vi "mcp&phosvol.vi"() -> ()   [LabVIEW 2014, in "Panels.lvlib"]
uses:
  Panels.lvlib
  CSlibraries-extern/DimLVEvent/DimIndicators/DimIndicators.lvlib
  CSCore/CSSystem/CoreLib/CoreLib.lvlib
  CSlibraries/UtilityLib/UtilityLib.valueStatus.ctl
  CSlibraries/UtilityLib/UtilityLib.lvlib
  CSlibraries-extern/DimLVEvent/LVDimInterface/LVDimInterface.lvlib
  Instance           1 19Saved   mcp&phosvol .vi
  CSlibraries-extern/DimLVEvent/DimIndicators/DimIndicators.numericArrayType.ctl
  CSlibraries-extern/DimLVEvent/DimIndicators/DimIndicators.anyType.ctl
  CSlibraries-extern/DimLVEvent/DimIndicators/DimIndicators.numericType.ctl
panel:
  in  "MPC_Collector_SetValueInfoData":T1={"data"=[0.0, 2200.0, -1.0], "no link"=FALSE, "quality"=0, "timeStamp"=3270208308.169}
  in  "CEM_Plate_SetValueInfoData":T1={"data"=[0.0, 2200.0, -1.0], "no link"=FALSE, "quality"=0, "timeStamp"=3270208308.169}
  in  "MPC_Collector_SetData":T1={"data"=[0.0, 0.0, 0.0, 0.0], "no link"=FALSE, "quality"=1, "timeStamp"=3270208307.575}
  in  "CEM_Plate_SetData":T1={"data"=[0.0, 0.0, 0.0, 0.0], "no link"=FALSE, "quality"=1, "timeStamp"=3270208307.575}
  in  "Daly_Collector_MonData":T2={"data"=inf, "no link"=FALSE, "quality"=1, "timeStamp"=3270208308.169}
  in  "CEM_Plate_MonData":T2={"data"=inf, "no link"=FALSE, "quality"=1, "timeStamp"=3270208308.169}
  in  "Daly_Collector":bool
  out "Daly_Collector_Mon":dbl=inf format="%.4f"
  in  "CEM_Plate":bool
  out "CEM_Plate_Mon":dbl=inf format="%.4f"
  in  "BOB3_PHO_SetValueInfoData":T1={"data"=[0.0, 2000.0, -1.0], "no link"=FALSE, "quality"=0, "timeStamp"=3270208308.169}
  in  "SetFileLocation_Data":T3={"data"="NOLINK", "no link"=TRUE, "quality"=-1, "timeStamp"=0.0}
  in  "BOB1_MCP":bool
  in  "BOB1_Pho":bool
  in  "BOB6MCPin_MonData":T2={"data"=32767.0, "no link"=FALSE, "quality"=1, "timeStamp"=3270208308.169}
  in  "BOB3MCPout_MonData":T2={"data"=32767.0, "no link"=FALSE, "quality"=1, "timeStamp"=3270208308.169}
  in  "BOB1BETAout_MonData":T2={"data"=32767.0, "no link"=FALSE, "quality"=1, "timeStamp"=3270208308.169}
  in  "BOB2MCPin_MonData":T2={"data"=32767.0, "no link"=FALSE, "quality"=1, "timeStamp"=3270208308.169}
  in  "BOB1BETAin_MonData":T2={"data"=32767.0, "no link"=FALSE, "quality"=1, "timeStamp"=3270208308.153}
  in  "BOB2MCPout_MonData":T2={"data"=32767.0, "no link"=FALSE, "quality"=1, "timeStamp"=3270208308.153}
  in  "BOB3MCPin_MonData":T2={"data"=32767.0, "no link"=FALSE, "quality"=1, "timeStamp"=3270208308.169}
  in  "BOB6MCPout_MonData":T2={"data"=32767.0, "no link"=FALSE, "quality"=1, "timeStamp"=3270208308.169}
  in  "BOB5MCPin_MonData":T2={"data"=32767.0, "no link"=FALSE, "quality"=1, "timeStamp"=3270208308.169}
  in  "BOB5MCPout_MonData":T2={"data"=32767.0, "no link"=FALSE, "quality"=1, "timeStamp"=3270208308.169}
  in  "BOB4MCPin_MonData":T2={"data"=32767.0, "no link"=FALSE, "quality"=1, "timeStamp"=3270208308.169}
  in  "BOB4MCPout_MonData":T2={"data"=32767.0, "no link"=FALSE, "quality"=1, "timeStamp"=3270208308.169}
  out "BOB6MCPin_Mon":bool
  out "BOB6MCPout_Mon":bool
  out "BOB5MCPin_Mon":bool
  out "BOB5MCPout_Mon":bool
  out "BOB4MCPin_Mon":bool
  out "BOB4MCPin_Mon":bool
  out "BOB3MCPin_Mon":bool
  out "BOB3MCPout_Mon":bool
  out "BOB2MCPin_Mon":bool
  out "BOB2MCPout_Mon":bool
  out "BOB1BETAin_Mon":bool
  out "BOB1BETAout_Mon":bool
  in  "SetFileLocation":path=path "\\\\intranet\\Files/projects/lebit/Data Exchange/data/MCP&PhosVolControl"
  in  "BOB6_MCP_SetValueInfoData":T1={"data"=[0.0, 2200.0, -1.0], "no link"=FALSE, "quality"=0, "timeStamp"=3270208308.169}
  in  "BOB6_MCP_SetData":T1={"data"=[0.0, 0.0, 0.0, 0.0], "no link"=FALSE, "quality"=1, "timeStamp"=3270208307.575}
  in  "BOB6_MCP_MonData":T2={"data"=inf, "no link"=FALSE, "quality"=1, "timeStamp"=3270208308.169}
  in  "BOB6_MCP":bool
  in  "BOB6_Pho":bool
  in  "BOB5_MCP":bool
  in  "BOB5_Pho":bool
  in  "BOB3_MCP":bool
  in  "BOB3_Pho":bool
  in  "BOB6_Pho_SetValueInfoData":T1={"data"=[0.0, 3000.0, -1.0], "no link"=FALSE, "quality"=0, "timeStamp"=3270208308.169}
  in  "BOB6_Pho_SetData":T1={"data"=[0.0, 0.0, 0.0, 0.0], "no link"=FALSE, "quality"=1, "timeStamp"=3270208307.575}
  in  "BOB6_Pho_MonData":T2={"data"=inf, "no link"=FALSE, "quality"=1, "timeStamp"=3270208308.169}
  out "BOB2_MCP_Mon":dbl=inf format="%.4f"
  out "BOB1_MCP_Mon":dbl=inf format="%.4f"
  out "i ref out":refnum<vi>
  in  "Last Loaded File_Data":T3={"data"="NOLINK", "no link"=TRUE, "quality"=-1, "timeStamp"=0.0}
  out "FileUpToDate":bool=TRUE caption="Parameter Changed"
  in  "BOB1_MCP_SetValueInfoData":T1={"data"=[0.0, 10.0, -1.0], "no link"=FALSE, "quality"=0, "timeStamp"=3270208308.153}
  in  "BOB2_Pho_SetValueInfoData":T1={"data"=[0.0, 3000.0, -1.0], "no link"=FALSE, "quality"=0, "timeStamp"=3270208308.169}
  in  "BOB2_MCP_SetValueInfoData":T1={"data"=[0.0, 10.0, -1.0], "no link"=FALSE, "quality"=0, "timeStamp"=3270208308.169}
  in  "BOB3_MCP_SetValueInfoData":T1={"data"=[0.0, 2000.0, -1.0], "no link"=FALSE, "quality"=0, "timeStamp"=3270208308.169}
  in  "BOB4_Pho_SetValueInfoData":T1={"data"=[0.0, 3000.0, -1.0], "no link"=FALSE, "quality"=0, "timeStamp"=3270208308.169}
  in  "BOB4_MCP_SetValueInfoData":T1={"data"=[0.0, 2000.0, -1.0], "no link"=FALSE, "quality"=0, "timeStamp"=3270208308.169}
  in  "BOB5_Pho_SetValueInfoData":T1={"data"=[0.0, 3000.0, -1.0], "no link"=FALSE, "quality"=0, "timeStamp"=3270208308.153}
  in  "BOB5_MCP_SetValueInfoData":T1={"data"=[0.0, 2000.0, -1.0], "no link"=FALSE, "quality"=0, "timeStamp"=3270208308.169}
  in  "BOB1_Pho_SetValueInfoData":T1={"data"=[0.0, 10.0, -1.0], "no link"=FALSE, "quality"=0, "timeStamp"=3270208308.169}
  in  "BOB1_Pho_SetData":T1={"data"=[0.0, 0.0, 0.0, 0.0], "no link"=FALSE, "quality"=1, "timeStamp"=3270208307.575}
  in  "BOB5_Pho_SetData":T1={"data"=[0.0, 0.0, 0.0, 0.0], "no link"=FALSE, "quality"=1, "timeStamp"=3270208307.575}
  in  "BOB4_MCP_SetData":T1={"data"=[0.0, 0.0, 0.0, 0.0], "no link"=FALSE, "quality"=1, "timeStamp"=3270208307.575}
  in  "BOB4_Pho_SetData":T1={"data"=[0.0, 0.0, 0.0, 0.0], "no link"=FALSE, "quality"=1, "timeStamp"=3270208307.575}
  in  "BOB3_MCP_SetData":T1={"data"=[0.0, 0.0, 0.0, 0.0], "no link"=FALSE, "quality"=1, "timeStamp"=3270208307.575}
  in  "BOB3_Pho_SetData":T1={"data"=[0.0, 0.0, 0.0, 0.0], "no link"=FALSE, "quality"=1, "timeStamp"=3270208307.591}
  in  "BOB2_MCP_SetData":T1={"data"=[0.0, 0.0, 0.0, 0.0], "no link"=FALSE, "quality"=1, "timeStamp"=3270208307.575}
  in  "BOB2_Pho_SetData":T1={"data"=[0.0, 0.0, 0.0, 0.0], "no link"=FALSE, "quality"=1, "timeStamp"=3270208307.575}
  in  "BOB1_MCP_SetData":T1={"data"=[0.0, 0.0, 0.0, 0.0], "no link"=FALSE, "quality"=1, "timeStamp"=3270208307.575}
  in  "BOB5_MCP_SetData":T1={"data"=[0.0, 0.0, 0.0, 0.0], "no link"=FALSE, "quality"=1, "timeStamp"=3270208307.575}
  out "Last Loaded File":string
  in  "BOB5_MCP_MonData":T2={"data"=inf, "no link"=FALSE, "quality"=1, "timeStamp"=3270208308.169}
  in  "BOB5_Pho_MonData":T2={"data"=inf, "no link"=FALSE, "quality"=1, "timeStamp"=3270208308.169}
  in  "BOB4_MCP_MonData":T2={"data"=inf, "no link"=FALSE, "quality"=1, "timeStamp"=3270208308.169}
  in  "BOB4_Pho_MonData":T2={"data"=inf, "no link"=FALSE, "quality"=1, "timeStamp"=3270208308.169}
  in  "BOB3_MCP_MonData":T2={"data"=inf, "no link"=FALSE, "quality"=1, "timeStamp"=3270208308.169}
  in  "BOB3_Pho_MonData":T2={"data"=inf, "no link"=FALSE, "quality"=1, "timeStamp"=3270208308.169}
  in  "BOB2_MCP_MonData":T2={"data"=inf, "no link"=FALSE, "quality"=1, "timeStamp"=3270208308.153}
  in  "BOB2_Pho_MonData":T2={"data"=inf, "no link"=FALSE, "quality"=1, "timeStamp"=3270208308.153}
  in  "BOB1_MCP_MonData":T2={"data"=inf, "no link"=FALSE, "quality"=1, "timeStamp"=3270208308.169}
  in  "BOB1_Pho_MonData":T2={"data"=inf, "no link"=FALSE, "quality"=1, "timeStamp"=3270208308.169}
  out "BOB3_MCP_Mon":dbl=inf format="%.4f"
  out "BOB2_Pho_Mon":dbl=inf format="%.4f"
  out "BOB6_MCP_Mon":dbl=inf format="%.4f"
  out "BOB4_Pho_Mon":dbl=inf format="%.4f"
  out "BOB3_Pho_Mon":dbl=inf format="%.4f"
  out "BOB1_Pho_Mon":dbl=inf format="%.4f"
  out "BOB5_Pho_Mon":dbl=inf format="%.4f"
  out "BOB4_MCP_Mon":dbl=inf format="%.4f"
  out "BOB5_MCP_Mon":dbl=inf format="%.4f"
  out "BOB6_Pho_Mon":dbl=inf format="%.4f"
  # "Parameter changed, data file is no longer up-to-date."
  # "BOB2_Pho"
  # "BOB4_Pho"
  # "BOB2_MCP"
  # "BOB4_MCP"
  # "IN"
  # "OUT"
  # "IN"
  # "OUT"
  # "IN"
  # "OUT"
  # "IN"
  # "OUT"
  # "IN"
  # "OUT"
  # "IN"
  # "OUT"
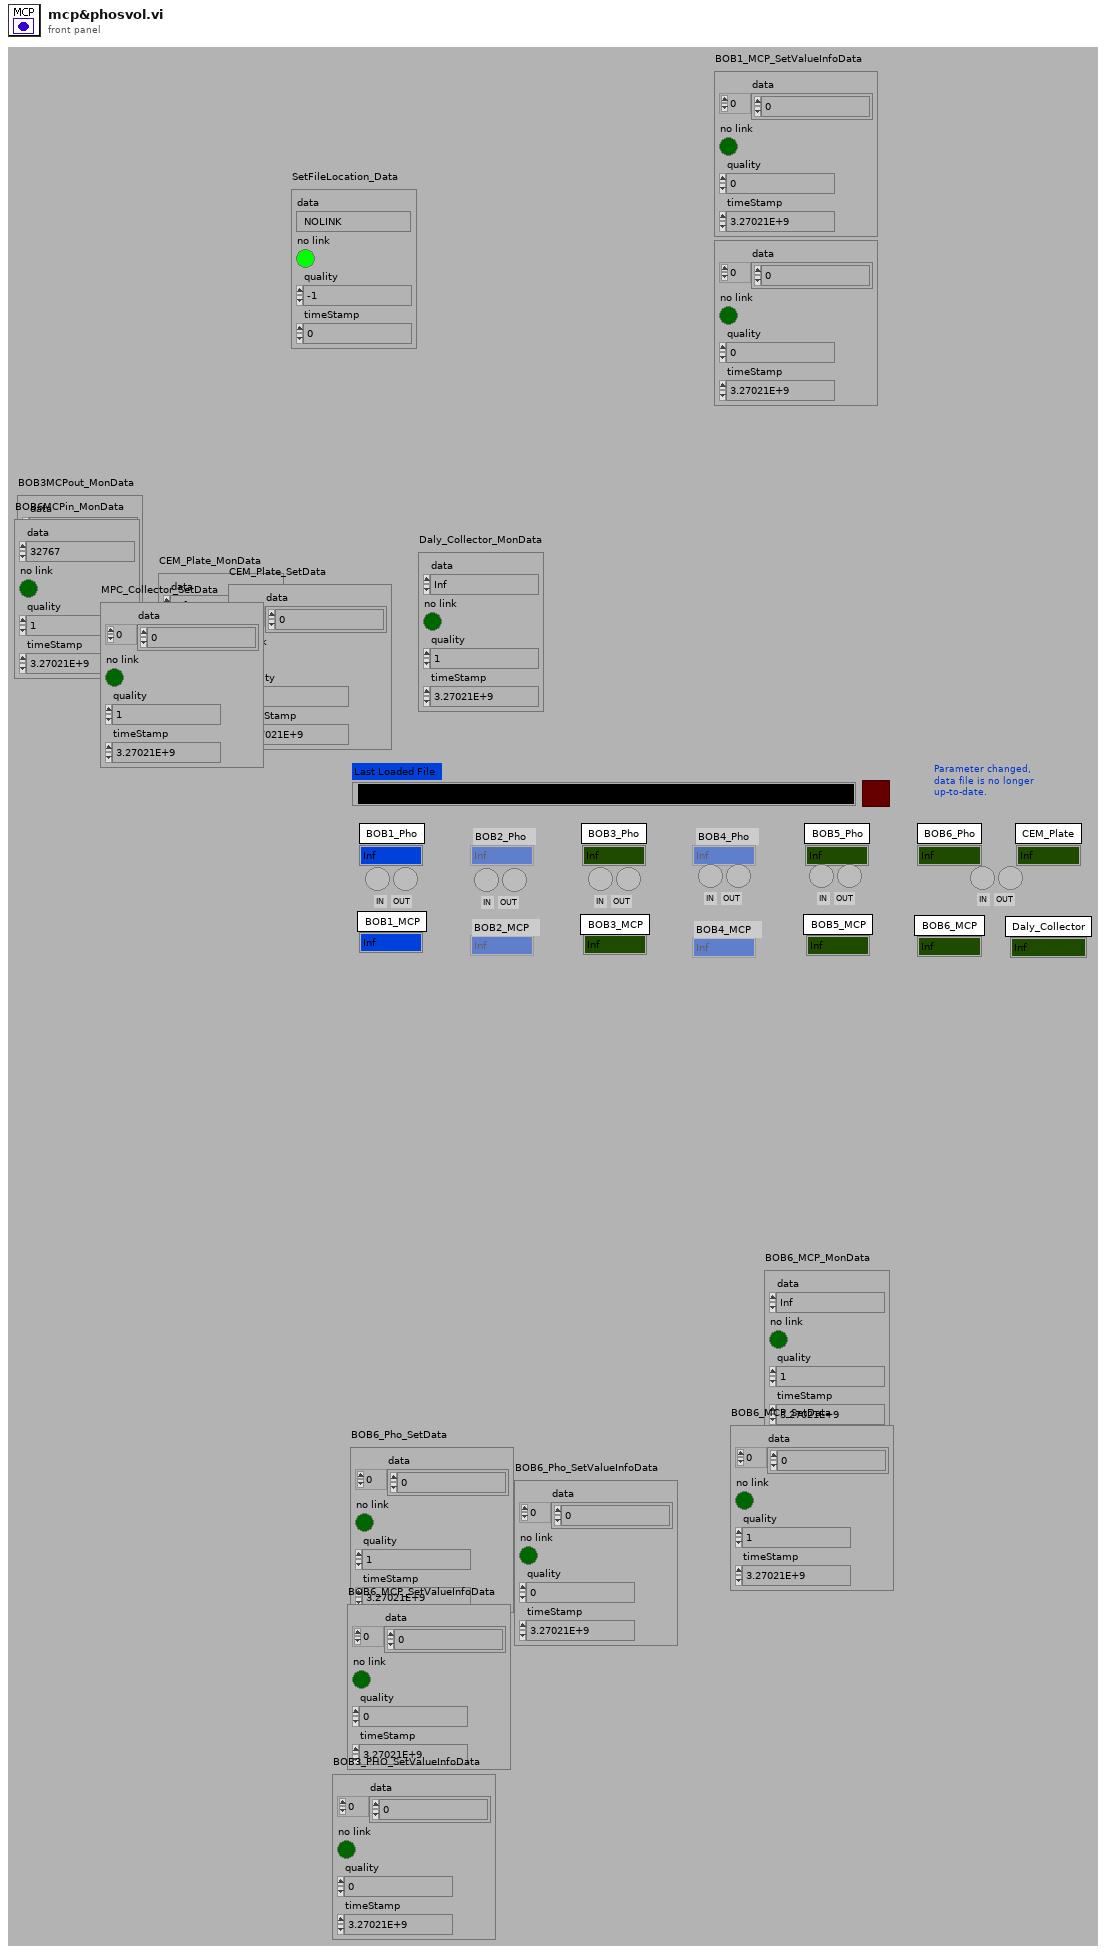
[diagram p1: front panel]
types:
  T1 = typedef "DimIndicators.lvlib/DimIndicators.numericArrayType.ctl" = cluster{"data":dbl[], "no link":bool, "quality":i32, "timeStamp":dbl}
  T2 = typedef "DimIndicators.lvlib/DimIndicators.numericType.ctl" = cluster{"data":dbl, "no link":bool, "quality":i32, "timeStamp":dbl}
  T3 = typedef "DimIndicators.lvlib/DimIndicators.anyType.ctl" = cluster{"data":string, "no link":bool, "quality":i32, "timeStamp":dbl}
  T4 = typedef "UtilityLib.lvlib/UtilityLib.valueStatus.ctl" = enum16{"no info available", "stand by/off", "on", "warning", "alarm/malfunction", "not implemented", "user action required", "important information", "system default", "control default", "indicator default", "button default"}
  T5 = cluster{"data":string, "no link":bool, "quality":i32, "timeStamp":dbl}
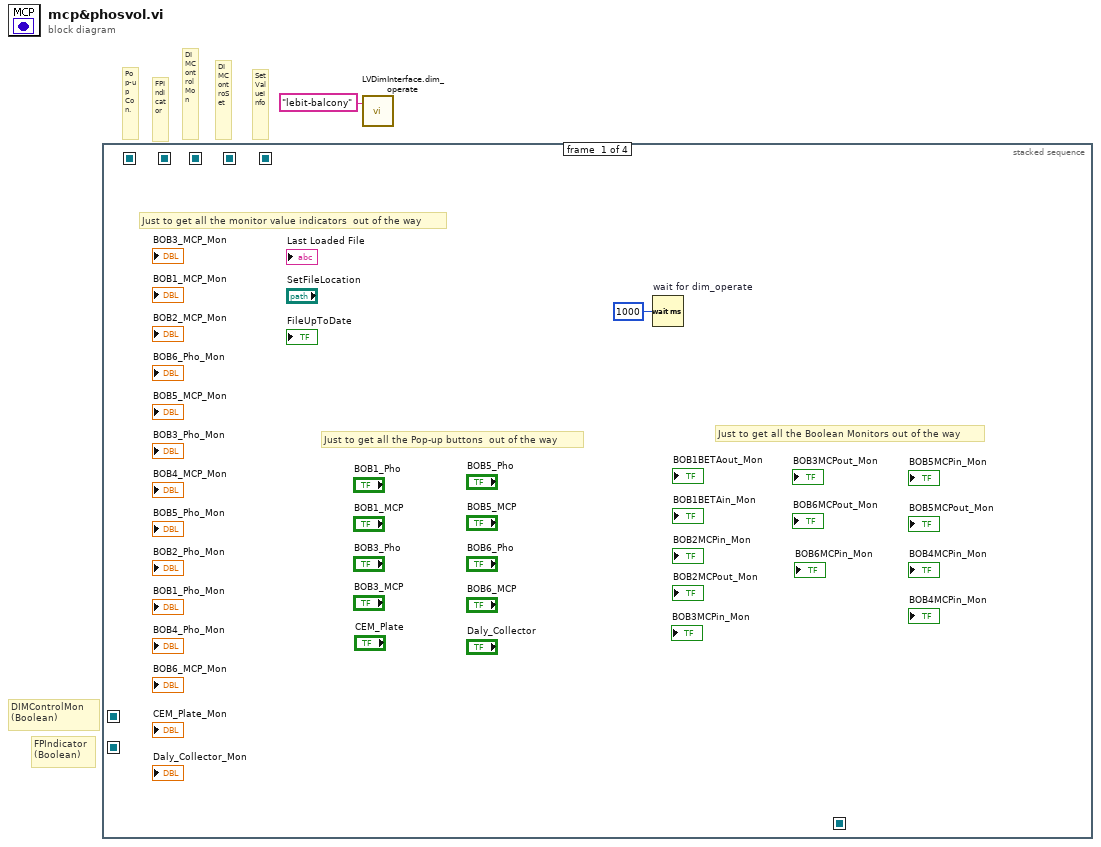
[diagram p0: block diagram]
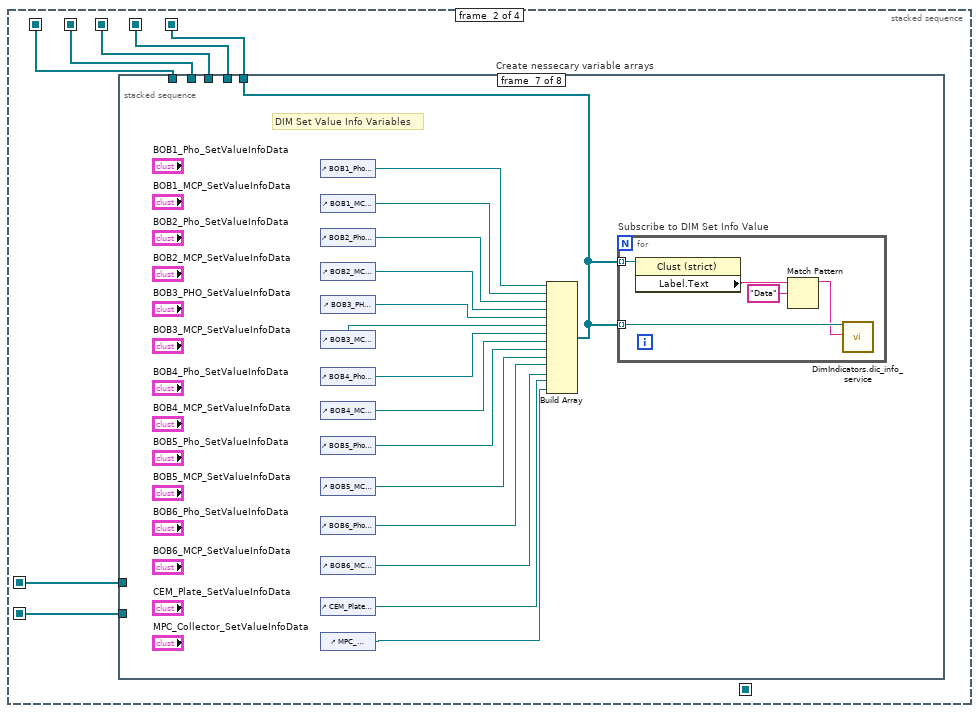
[diagram p2: hidden frame]
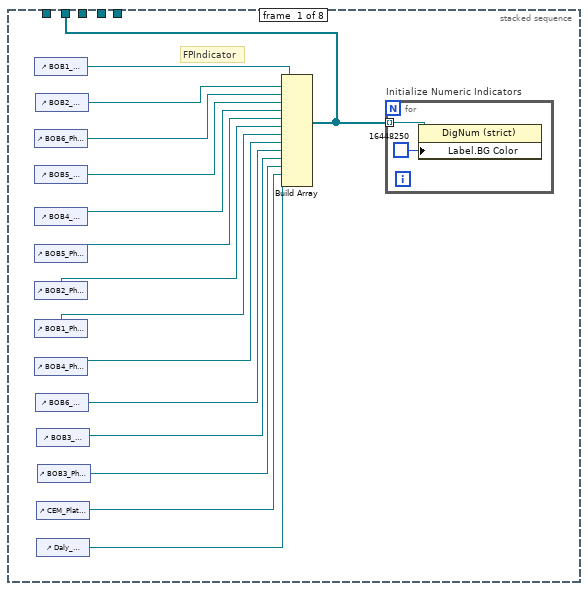
[diagram p3: hidden frame]
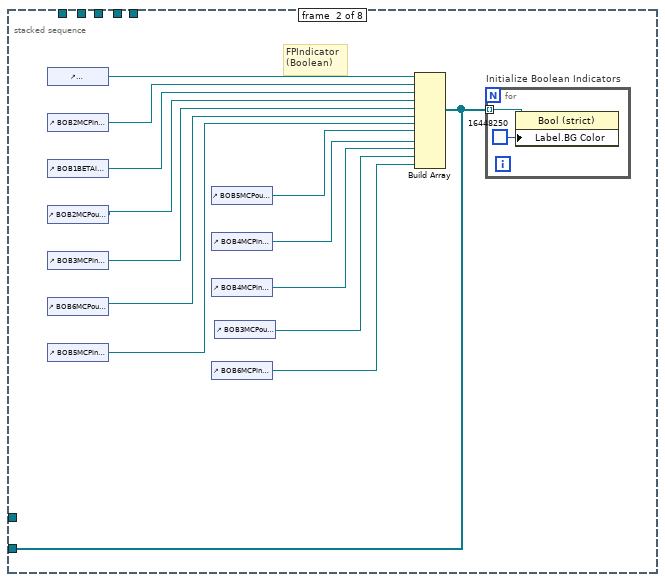
[diagram p4: hidden frame]
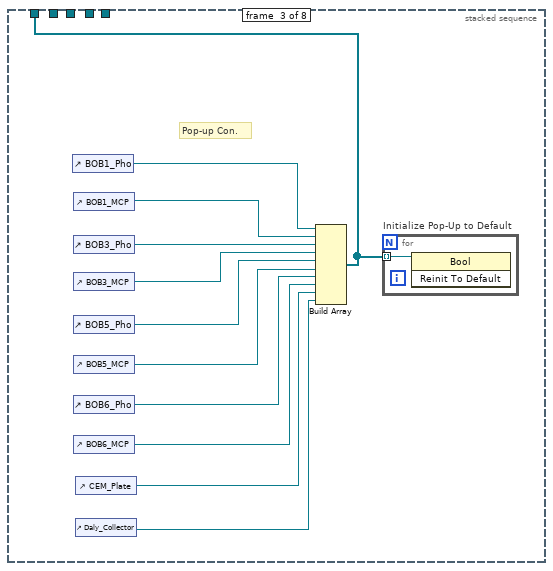
[diagram p5: hidden frame]
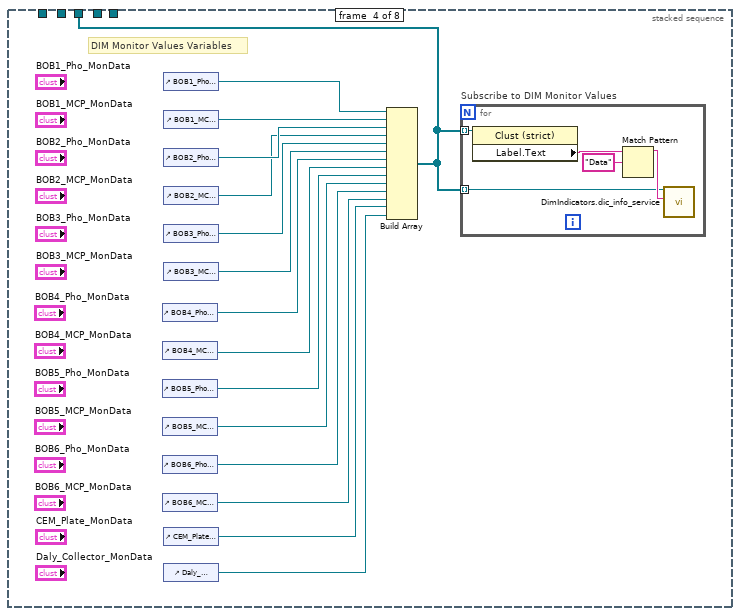
[diagram p6: hidden frame]
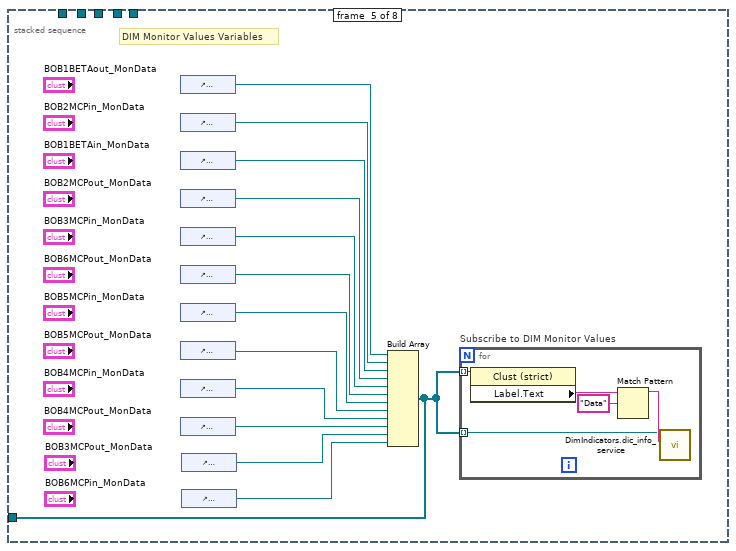
[diagram p7: hidden frame]
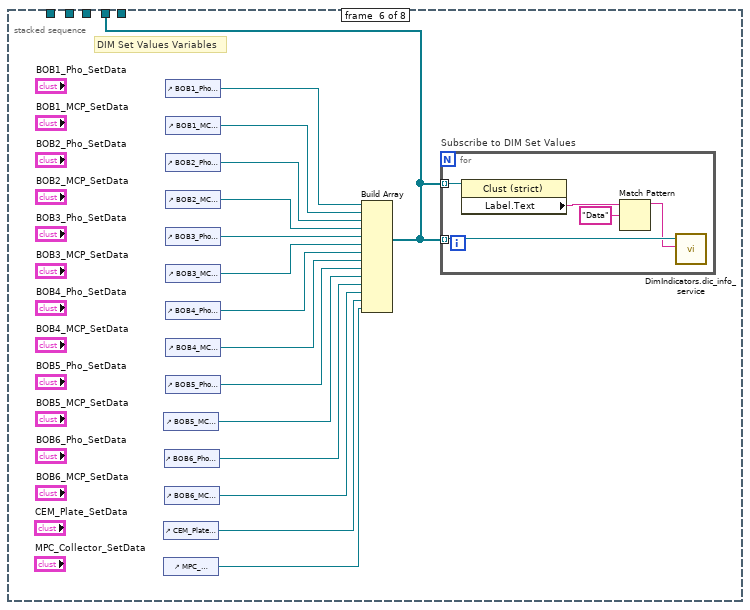
[diagram p8: hidden frame]
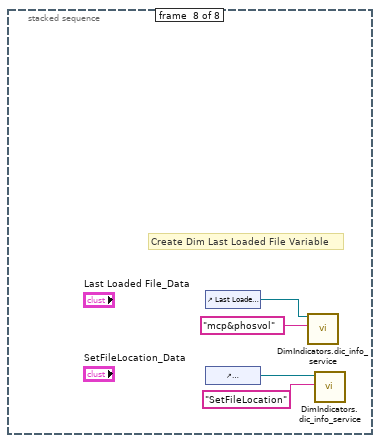
[diagram p9: hidden frame]
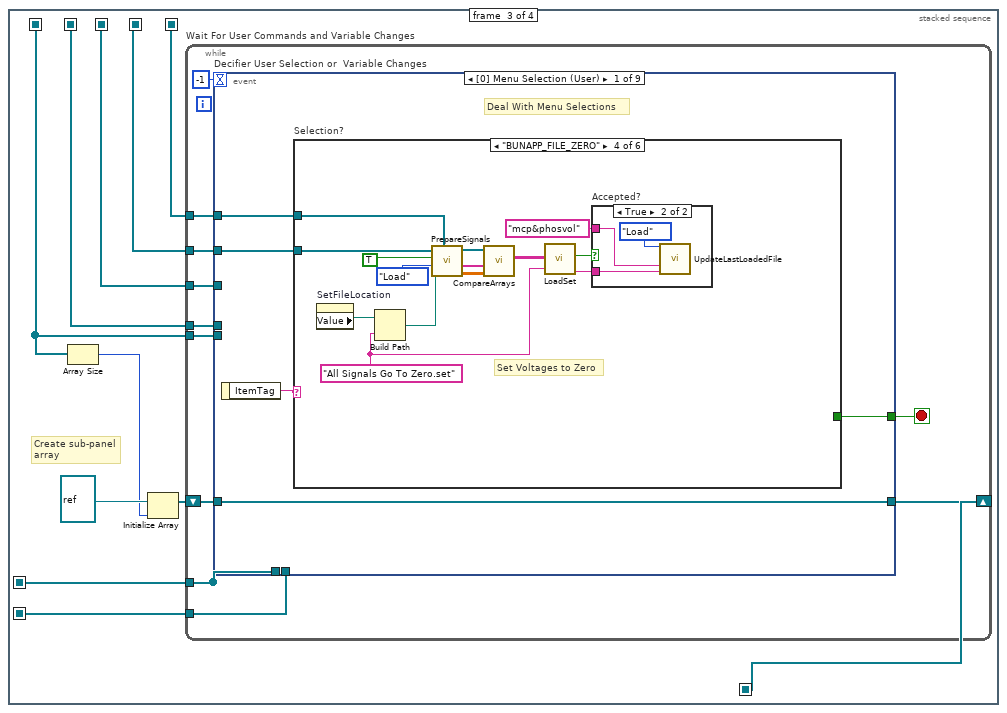
[diagram p10: hidden frame]
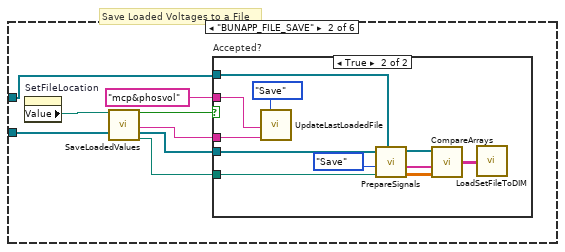
[diagram p12: hidden frame]
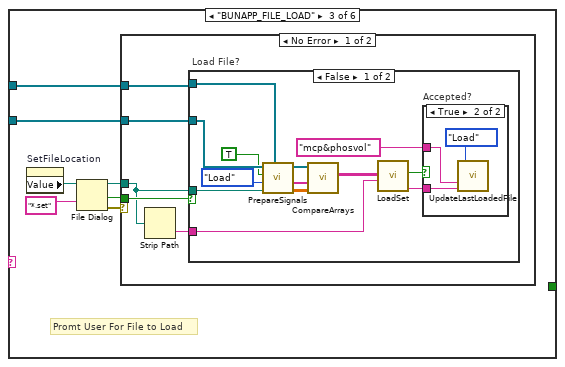
[diagram p14: hidden frame]
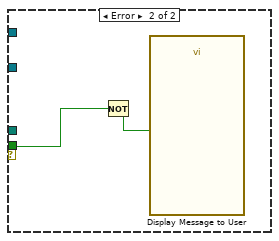
[diagram p17: hidden frame]
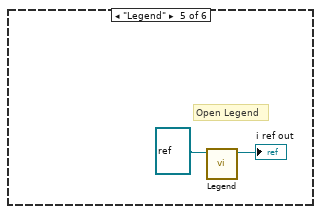
[diagram p19: hidden frame]
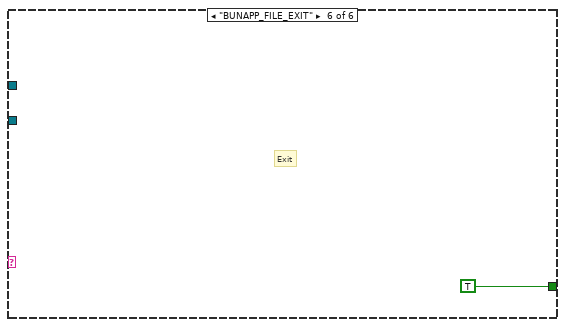
[diagram p20: hidden frame]
diagram:
  # "FPIndicator\n(Boolean)"
  # "DIMControlMon\n(Boolean)"
  # "Pop-up Con."
  # "SetValueInfo"
  # "DIMControSet"
  # "DIMControlMon"
  # "FPIndicator"
  n1 = stacked-sequence {
    seq-local: [_ w9 _ _] -> [_ _ w143 _]
    seq-local: [_ w4 _ _] -> [_ _ w146 w375]
    seq-local: [_ _ w141 _] -> [_ _ _ w374]
    seq-local: [_ w5 _ _] -> [_ _ w140 w373]
    seq-local: [_ w3 _ _] -> [_ _ w139 w372]
    seq-local: [_ w7 _ _] -> [_ _ w138 _]
    seq-local: [_ w8 _ _] -> [_ _ w136 _]
    seq-local: [_ w6 _ _] -> [_ _ w137 w371]
    frame #0 {
      # "Just to get all the Boolean Monitors out of the way"
      # "Just to get all the Pop-up buttons  out of the way"
      # "Just to get all the monitor value indicators  out of the way"
      n2 = Wait (ms) "wait for dim_operate"(milliseconds to wait=u32 1000) -> ()  [unwired: 1 out]
    }
    frame #1 {
      # "Arrange references to all monitor-value related buttons into an array."
      n3 = stacked-sequence "Create nessecary variable arrays" {
        tunnel: [w12 _ _ _ _ _ _ _] -> w9
        tunnel: [_ w27 _ _ _ _ _ _] -> w8
        tunnel: [_ _ w44 _ _ _ _ _] -> w7
        tunnel: [_ _ _ w56 _ _ _ _] -> w4
        tunnel: [_ _ _ _ w74 _ _ _] -> w6
        tunnel: [_ _ _ _ _ w94 _ _] -> w5
        tunnel: [_ _ _ _ _ _ w116 _] -> w3
        frame #0 {
          # "FPIndicator"
          n4 = control-ref of="BOB1_MCP_Mon"() -> (w18:refnum<vi>)
          n5 = control-ref of="BOB6_Pho_Mon"() -> (w15:refnum<vi>)
          n6 = control-ref of="BOB5_MCP_Mon"() -> (w16:refnum<vi>)
          n7 = control-ref of="BOB4_MCP_Mon"() -> (w24:refnum<vi>)
          n8 = control-ref of="BOB5_Pho_Mon"() -> (w23:refnum<vi>)
          n9 = control-ref of="BOB2_Pho_Mon"() -> (w22:refnum<vi>)
          n10 = control-ref of="BOB1_Pho_Mon"() -> (w21:refnum<vi>)
          n11 = control-ref of="BOB4_Pho_Mon"() -> (w20:refnum<vi>)
          n12 = control-ref of="BOB2_MCP_Mon"() -> (w14:refnum<vi>)
          n13 = control-ref of="BOB6_MCP_Mon"() -> (w19:refnum<vi>)
          n14 = control-ref of="BOB3_MCP_Mon"() -> (w17:refnum<vi>)
          n15 = control-ref of="CEM_Plate_Mon"() -> (w11:refnum<vi>)
          n16 = control-ref of="Daly_Collector_Mon"() -> (w10:refnum<vi>)
          n17 = control-ref of="BOB3_Pho_Mon"() -> (w13:refnum<vi>)
          n18 = Build Array(w18, w14, w15, w16, w24, w23, w22, w21, w20, w19, w17, w13, w11, w10) -> (w12:refnum<vi>[])
          n19 = for "Initialize Numeric Indicators" {
            tunnel: w12 -> [w26] mode=indexing
            n20 = property class="DigNum (strict)"(reference=w26, "Label.BG Color"=u32 16448250 ("Color Box")) -> ()  [unwired: 1 in, 2 out]
          }
        }
        frame #1 {
          # "FPIndicator\n(Boolean)"
          n21 = control-ref of="BOB1BETAout_Mon"() -> (w39:refnum<vi>)
          n22 = control-ref of="BOB2MCPin_Mon"() -> (w38:refnum<vi>)
          n23 = control-ref of="BOB1BETAin_Mon"() -> (w37:refnum<vi>)
          n24 = control-ref of="BOB2MCPout_Mon"() -> (w36:refnum<vi>)
          n25 = control-ref of="BOB3MCPin_Mon"() -> (w35:refnum<vi>)
          n26 = control-ref of="BOB6MCPout_Mon"() -> (w34:refnum<vi>)
          n27 = control-ref of="BOB5MCPin_Mon"() -> (w33:refnum<vi>)
          n28 = control-ref of="BOB5MCPout_Mon"() -> (w32:refnum<vi>)
          n29 = control-ref of="BOB4MCPin_Mon"() -> (w31:refnum<vi>)
          n30 = control-ref of="BOB4MCPin_Mon"() -> (w30:refnum<vi>)
          n31 = control-ref of="BOB6MCPin_Mon"() -> (w28:refnum<vi>)
          n32 = control-ref of="BOB3MCPout_Mon"() -> (w29:refnum<vi>)
          n33 = Build Array(w39, w38, w37, w36, w35, w34, w33, w32, w31, w30, w29, w28) -> (w27:refnum<vi>[])
          n34 = for "Initialize Boolean Indicators" {
            tunnel: w27 -> [w41] mode=indexing
            n35 = property class="Bool (strict)"(reference=w41, "Label.BG Color"=u32 16448250 ("Color Box")) -> ()  [unwired: 1 in, 2 out]
          }
        }
        frame #2 {
          # "Pop-up Con."
          n36 = control-ref of="BOB1_Pho"() -> (w46:refnum<vi>)
          n37 = control-ref of="BOB1_MCP"() -> (w45:refnum<vi>)
          n38 = control-ref of="BOB3_Pho"() -> (w52:refnum<vi>)
          n39 = control-ref of="BOB3_MCP"() -> (w51:refnum<vi>)
          n40 = control-ref of="BOB5_Pho"() -> (w50:refnum<vi>)
          n41 = control-ref of="BOB5_MCP"() -> (w49:refnum<vi>)
          n42 = control-ref of="BOB6_Pho"() -> (w48:refnum<vi>)
          n43 = control-ref of="BOB6_MCP"() -> (w47:refnum<vi>)
          n44 = control-ref of="CEM_Plate"() -> (w43:refnum<vi>)
          n45 = control-ref of="Daly_Collector"() -> (w42:refnum<vi>)
          n46 = Build Array(w46, w45, w52, w51, w50, w49, w48, w47, w43, w42) -> (w44:refnum<vi>[])
          n47 = for "Initialize Pop-Up to Default" {
            tunnel: w44 -> [w53] mode=indexing
            n48 = invoke class="Bool" method="Reinit To Default"(reference=w53) -> ()  [unwired: 2 in, 3 out]
          }
        }
        frame #3 {
          # "DIM Monitor Values Variables"
          n49 = control-ref of="BOB4_Pho_MonData"() -> (w62:refnum<vi>)
          n50 = control-ref of="BOB4_MCP_MonData"() -> (w60:refnum<vi>)
          n51 = control-ref of="BOB5_Pho_MonData"() -> (w59:refnum<vi>)
          n52 = control-ref of="BOB5_MCP_MonData"() -> (w58:refnum<vi>)
          n53 = control-ref of="BOB6_Pho_MonData"() -> (w61:refnum<vi>)
          n54 = control-ref of="BOB6_MCP_MonData"() -> (w57:refnum<vi>)
          n55 = control-ref of="BOB1_Pho_MonData"() -> (w68:refnum<vi>)
          n56 = control-ref of="BOB1_MCP_MonData"() -> (w67:refnum<vi>)
          n57 = control-ref of="BOB2_Pho_MonData"() -> (w66:refnum<vi>)
          n58 = control-ref of="BOB2_MCP_MonData"() -> (w65:refnum<vi>)
          n59 = control-ref of="BOB3_Pho_MonData"() -> (w64:refnum<vi>)
          n60 = control-ref of="BOB3_MCP_MonData"() -> (w63:refnum<vi>)
          n61 = control-ref of="CEM_Plate_MonData"() -> (w55:refnum<vi>)
          n62 = control-ref of="Daly_Collector_MonData"() -> (w54:refnum<vi>)
          n63 = Build Array(w68, w67, w66, w65, w64, w63, w62, w60, w59, w58, w61, w57, w55, w54) -> (w56:refnum<vi>[])
          n64 = for "Subscribe to DIM Monitor Values" {
            tunnel: w56 -> [w70] mode=indexing
            tunnel: w56 -> [w69] mode=indexing
            n65 = property class="Clust (strict)"(reference=w69) -> ("Label.Text"=w72:string)  [unwired: 1 in, 2 out]
            n66 = Match Pattern(string=w72, regular expression="Data") -> (before substring=w71:string)  [unwired: 1 in, 3 out]
            n67 = call "DimIndicators.dic_info_service.vi"("controlRef"=w70, "serviceName"=w71) -> ()  [unwired: 16 in, 2 out]
          }
        }
        frame #4 {
          # "DIM Monitor Values Variables"
          n68 = control-ref of="BOB1BETAout_MonData"() -> (w86:refnum<vi>)
          n69 = control-ref of="BOB2MCPin_MonData"() -> (w85:refnum<vi>)
          n70 = control-ref of="BOB1BETAin_MonData"() -> (w84:refnum<vi>)
          n71 = control-ref of="BOB2MCPout_MonData"() -> (w83:refnum<vi>)
          n72 = control-ref of="BOB3MCPin_MonData"() -> (w82:refnum<vi>)
          n73 = control-ref of="BOB6MCPout_MonData"() -> (w81:refnum<vi>)
          n74 = control-ref of="BOB5MCPin_MonData"() -> (w80:refnum<vi>)
          n75 = control-ref of="BOB5MCPout_MonData"() -> (w79:refnum<vi>)
          n76 = control-ref of="BOB4MCPin_MonData"() -> (w78:refnum<vi>)
          n77 = control-ref of="BOB4MCPout_MonData"() -> (w77:refnum<vi>)
          n78 = control-ref of="BOB3MCPout_MonData"() -> (w76:refnum<vi>)
          n79 = control-ref of="BOB6MCPin_MonData"() -> (w75:refnum<vi>)
          n80 = Build Array(w86, w85, w84, w83, w82, w81, w80, w79, w78, w77, w76, w75) -> (w74:refnum<vi>[])
          n81 = for "Subscribe to DIM Monitor Values" {
            tunnel: w74 -> [w88] mode=indexing
            tunnel: w74 -> [w87] mode=indexing
            n82 = property class="Clust (strict)"(reference=w87) -> ("Label.Text"=w90:string)  [unwired: 1 in, 2 out]
            n83 = Match Pattern(string=w90, regular expression="Data") -> (before substring=w89:string)  [unwired: 1 in, 3 out]
            n84 = call "DimIndicators.dic_info_service.vi"("controlRef"=w88, "serviceName"=w89) -> ()  [unwired: 16 in, 2 out]
          }
        }
        frame #5 {
          # "DIM Set Values Variables"
          n85 = control-ref of="BOB5_MCP_SetData"() -> (w97:refnum<vi>)
          n86 = control-ref of="CEM_Plate_SetData"() -> (w93:refnum<vi>)
          n87 = control-ref of="MPC_Collector_SetData"() -> (w92:refnum<vi>)
          n88 = control-ref of="BOB6_Pho_SetData"() -> (w96:refnum<vi>)
          n89 = control-ref of="BOB6_MCP_SetData"() -> (w95:refnum<vi>)
          n90 = control-ref of="BOB1_Pho_SetData"() -> (w106:refnum<vi>)
          n91 = control-ref of="BOB1_MCP_SetData"() -> (w105:refnum<vi>)
          n92 = control-ref of="BOB2_Pho_SetData"() -> (w104:refnum<vi>)
          n93 = control-ref of="BOB2_MCP_SetData"() -> (w103:refnum<vi>)
          n94 = control-ref of="BOB3_Pho_SetData"() -> (w102:refnum<vi>)
          n95 = control-ref of="BOB3_MCP_SetData"() -> (w101:refnum<vi>)
          n96 = control-ref of="BOB4_Pho_SetData"() -> (w100:refnum<vi>)
          n97 = control-ref of="BOB4_MCP_SetData"() -> (w99:refnum<vi>)
          n98 = control-ref of="BOB5_Pho_SetData"() -> (w98:refnum<vi>)
          n99 = Build Array(w106, w105, w104, w103, w102, w101, w100, w99, w98, w97, w96, w95, w93, w92) -> (w94:refnum<vi>[])
          n100 = for "Subscribe to DIM Set Values" {
            tunnel: w94 -> [w107] mode=indexing
            tunnel: w94 -> [w111] mode=indexing
            n101 = property class="Clust (strict)"(reference=w107) -> ("Label.Text"=w110:string)  [unwired: 1 in, 2 out]
            n102 = Match Pattern(string=w110, regular expression="Data") -> (before substring=w108:string)  [unwired: 1 in, 3 out]
            n103 = call "DimIndicators.dic_info_service.vi"("controlRef"=w111, "serviceName"=w108) -> ()  [unwired: 16 in, 2 out]
          }
        }
        frame #6 {
          # "DIM Set Value Info Variables"
          n104 = control-ref of="BOB1_Pho_SetValueInfoData"() -> (w126:refnum<vi>)
          n105 = control-ref of="BOB1_MCP_SetValueInfoData"() -> (w125:refnum<vi>)
          n106 = control-ref of="BOB2_Pho_SetValueInfoData"() -> (w124:refnum<vi>)
          n107 = control-ref of="BOB2_MCP_SetValueInfoData"() -> (w123:refnum<vi>)
          n108 = control-ref of="BOB3_PHO_SetValueInfoData"() -> (w114:refnum<vi>)
          n109 = control-ref of="BOB3_MCP_SetValueInfoData"() -> (w115:refnum<vi>)
          n110 = control-ref of="BOB4_Pho_SetValueInfoData"() -> (w122:refnum<vi>)
          n111 = control-ref of="BOB4_MCP_SetValueInfoData"() -> (w121:refnum<vi>)
          n112 = control-ref of="BOB5_Pho_SetValueInfoData"() -> (w120:refnum<vi>)
          n113 = control-ref of="BOB5_MCP_SetValueInfoData"() -> (w119:refnum<vi>)
          n114 = control-ref of="BOB6_Pho_SetValueInfoData"() -> (w118:refnum<vi>)
          n115 = control-ref of="BOB6_MCP_SetValueInfoData"() -> (w117:refnum<vi>)
          n116 = control-ref of="CEM_Plate_SetValueInfoData"() -> (w113:refnum<vi>)
          n117 = control-ref of="MPC_Collector_SetValueInfoData"() -> (w112:refnum<vi>)
          n118 = Build Array(w126, w125, w124, w123, w114, w115, w122, w121, w120, w119, w118, w117, w113, w112) -> (w116:refnum<vi>[])
          n119 = for "Subscribe to DIM Set Info Value" {
            tunnel: w116 -> [w127] mode=indexing
            tunnel: w116 -> [w131] mode=indexing
            n120 = property class="Clust (strict)"(reference=w127) -> ("Label.Text"=w130:string)  [unwired: 1 in, 2 out]
            n121 = Match Pattern(string=w130, regular expression="Data") -> (before substring=w128:string)  [unwired: 1 in, 3 out]
            n122 = call "DimIndicators.dic_info_service.vi"("controlRef"=w131, "serviceName"=w128) -> ()  [unwired: 16 in, 2 out]
          }
        }
        frame #7 {
          # "Create Dim Last Loaded File Variable"
          n123 = control-ref of="Last Loaded File_Data"() -> (w134:refnum<vi>)
          n124 = control-ref of="SetFileLocation_Data"() -> (w133:refnum<vi>)
          n125 = call "DimIndicators.dic_info_service.vi"("controlRef"=w134, "serviceName"="mcp&phosvol" ("string")) -> ()  [unwired: 16 in, 2 out]
          n126 = call "DimIndicators.dic_info_service.vi"("controlRef"=w133, "serviceName"="SetFileLocation") -> ()  [unwired: 16 in, 2 out]
        }
      }
    }
    frame #2 {
      # "Create sub-panel\narray"
      n127 = Array Size(array=w138) -> (size(s)=w142:i32)
      n128 = Initialize Array(refnum<vi> refnum ("vi reference"), w142) -> (w145:refnum<vi>[])
      n129 = while "Wait For User Commands and Variable Changes" {
        tunnel: w146 -> [w156]
        tunnel: w143 -> [w155]
        shift-right: [w153] -> w141
        shift-left: w145 -> [w154]
        tunnel: w140 -> [w152]
        tunnel: w139 -> [w151]
        tunnel: w138 -> [w149]
        tunnel: [w148] -> _
        tunnel: w137 -> [w148]
        tunnel: w136 -> [w147]
        stop <- w157 stop-if-true
        n130 = event "Decifier User Selection or  Variable Changes" shown="[0] Menu Selection (User)" {
          selector: _ -> [_ _ _ _ _ _ _ _ _]
          dyn-events: _ -> [_ _ _ _ _ _ _ _ _]
          timeout: -1 -> [_ _ _ _ _ _ _ _ _]
          tunnel: [w159 _ _ _ _ _ _ _ TRUE ("stop")] -> w157
          tunnel: w156 -> [_ _ _ _ _ _ _ _ w343]
          tunnel: w155 -> [_ _ _ w269 _ _ _ _ _]
          tunnel: w154 -> [w162 w235 w266 w268 w294 w327 w335 w340 w341]
          tunnel: [w162 w235 w266 w268 w294 w327 w333 w340 _] -> w153
          tunnel: w152 -> [w160 w233 w263 _ _ w324 _ _ w344]
          tunnel: w151 -> [w158 w232 w260 _ _ _ _ _ w345]
          tunnel: w149 -> [_ _ _ _ _ _ w329 _ _]
          tunnel: w148 -> [_ _ _ _ _ _ _ _ w342]
          tunnel: w147 -> [_ _ _ _ w292 _ _ _ _]
          event Menu Selection (User) {
            # "Deal With Menu Selections"
            n131 = event-data() -> ("ItemTag"=w161:string)  [unwired: 1 in]
            n132 = case "Selection?" shown="\"BUNAPP_FILE_ZERO\"" w161 {
              tunnel: w160 -> [_ w167 w187 w225 _ _]
              tunnel: [_ _ _ _ _ TRUE ("stop")] -> w159
              tunnel: w158 -> [_ w163 w182 w212 _ _]
              frame "False", Default {
              }
              frame "BUNAPP_FILE_SAVE" {
                # "Save Loaded Voltages to a File"
                n133 = property on="SetFileLocation" class="Path"() -> ("Value"=w168:path)  [unwired: 2 in, 2 out]
                n134 = call "SaveLoadedValues.vi"("Panel Location?"=w168, "DIMControlSet in"=w167) -> ("File Saved?"=w169:bool, "File Name"=w166:string, "DIMControlSet out"=w164:refnum<vi>[], "Path"=w165:path)  [unwired: 14 in]
                n135 = case "Accepted?" shown="True" w169 {
                  tunnel: w166 -> [_ w179]
                  tunnel: "mcp&phosvol" ("string") -> [_ w181]
                  tunnel: w164 -> [_ w180]
                  tunnel: w165 -> [_ w178]
                  tunnel: w163 -> [_ w172]
                  frame False {
                  }
                  frame True {
                    n136 = call "UpdateLastLoadedFile.vi"("LoadOrSave"=enum16{"Load", "Save"}."Save", "GUIName"=w181, "FileNameIn"=w179) -> ()  [unwired: 13 in]
                    n137 = call "PrepareSignals.vi"("SetValueInfo in"=w172, "setfile path"=w178, "Enum"=enum16{"Save", "Load"}."Save", "DIMControSet in"=w180) -> ("indexed loaded Array"=w176:dbl[][], "Name Array"=w177:string[], "DIMControSet out"=w175:refnum<vi>[])  [unwired: 5 in]
                    n138 = call "CompareArrays.vi"("indexed loaded Array"=w176, "Name Array"=w177, "DIMControSet"=w175) -> ("Table for loading values"=w174:string[][])  [unwired: 4 in]
                    n139 = call "LoadSetFileToDIM.vi"("output array"=w174) -> ()  [unwired: 2 in]
                  }
                }
              }
              frame "BUNAPP_FILE_LOAD" {
                # "Promt User For File to Load"
                n140 = property on="SetFileLocation" class="Path"() -> ("Value"=w184:path)  [unwired: 2 in, 2 out]
                n141 = File Dialog(6:"*.set" ("pattern (all files)"), 11:w184) -> (0:w183:errorcluster, 1:w188:bool, 3:w185:path)  [unwired: 5 in, 1 out]
                n142 = case shown="No Error" w183 {
                  tunnel: w188 -> [w193 w210]
                  tunnel: w187 -> [w192 _]
                  tunnel: w185 -> [w190 _]
                  tunnel: w182 -> [w189 _]
                  frame No Error {
                    n143 = Strip Path(path=w190) -> (name=w191:string)  [unwired: 1 out]
                    n144 = case "Load File?" shown="False" w193 {
                      tunnel: w192 -> [w206 _]
                      tunnel: w191 -> [w200 _]
                      tunnel: w190 -> [w201 _]
                      tunnel: w189 -> [w194 _]
                      frame False {
                        n145 = call "PrepareSignals.vi"("SetValueInfo in"=w194, "setfile path"=w201, "Enum"=enum16{"Save", "Load"}."Load", "Display Message to \nUser"=TRUE ("Display Message to \nUser"), "DIMControSet in"=w206) -> ("indexed loaded Array"=w204:dbl[][], "Name Array"=w203:string[], "DIMControSet out"=w205:refnum<vi>[])  [unwired: 4 in]
                        n146 = call "CompareArrays.vi"("indexed loaded Array"=w204, "Name Array"=w203, "DIMControSet"=w205) -> ("Table for loading values"=w202:string[][])  [unwired: 4 in]
                        n147 = call "LoadSet.vi"("File Name In"=w200, "output array"=w202) -> ("File Name out"=w199:string, "Accepted"=w198:bool)  [unwired: 8 in]
                        n148 = case "Accepted?" shown="True" w198 {
                          tunnel: w199 -> [_ w209]
                          tunnel: "mcp&phosvol" ("string") -> [_ w208]
                          frame False {
                          }
                          frame True {
                            n149 = call "UpdateLastLoadedFile.vi"("LoadOrSave"=enum16{"Load", "Save"}."Load", "GUIName"=w208, "FileNameIn"=w209) -> ()  [unwired: 13 in]
                          }
                        }
                      }
                      frame True {
                      }
                    }
                  }
                  frame Error {
                    n150 = Not(x=w210) -> (.not. x?=w211:bool)
                    n151 = call "Display Message to User"("Enable"=w211) -> ()  [unwired: 9 in, 2 out]
                  }
                }
              }
              frame "BUNAPP_FILE_ZERO" {
                w216 = "All Signals Go To Zero.set" ("File Name")
                # "Set Voltages to Zero"
                n152 = property on="SetFileLocation" class="Path"() -> ("Value"=w214:path)  [unwired: 2 in, 2 out]
                n153 = Build Path(base path=w214, name or relative path=w216) -> (appended path=w215:path)
                n154 = call "PrepareSignals.vi"("SetValueInfo in"=w212, "setfile path"=w215, "Enum"=enum16{"Save", "Load"}."Load", "Display Message to \nUser"=TRUE ("Display Message to \nUser"), "DIMControSet in"=w225) -> ("indexed loaded Array"=w223:dbl[][], "Name Array"=w222:string[], "DIMControSet out"=w224:refnum<vi>[])  [unwired: 4 in]
                n155 = call "CompareArrays.vi"("indexed loaded Array"=w223, "Name Array"=w222, "DIMControSet"=w224) -> ("Table for loading values"=w221:string[][])  [unwired: 4 in]
                n156 = call "LoadSet.vi"("File Name In"=w216, "output array"=w221) -> ("File Name out"=w219:string, "Accepted"=w220:bool)  [unwired: 8 in]
                n157 = case "Accepted?" shown="True" w220 {
                  tunnel: w219 -> [_ w228]
                  tunnel: "mcp&phosvol" ("string") -> [_ w227]
                  frame False {
                  }
                  frame True {
                    n158 = call "UpdateLastLoadedFile.vi"("LoadOrSave"=enum16{"Load", "Save"}."Load", "GUIName"=w227, "FileNameIn"=w228) -> ()  [unwired: 13 in]
                  }
                }
              }
              frame "Legend" {
                # "Open Legend"
                n159 = call "Legend.vi"("i ref in"=refnum<vi> refnum) -> ("i ref out"=→"i ref out":refnum<vi>)  [unwired: 10 in]
              }
              frame "BUNAPP_FILE_EXIT" {
                # "Exit"
              }
            }
          }
          event Value Change {
            n160 = event-data() -> ("NewVal"=w234:T3)  [unwired: 1 in]
            n161 = stacked-sequence "Update Set File Location and Last Loaded File" {
              tunnel: w234 -> [w237 _]
              tunnel: w233 -> [_ w255]
              tunnel: w232 -> [_ w253]
              frame #0 {
                # "Update Set File Location"
                n162 = Unbundle By Name(w237) -> ("data"=w246:string, "no link"=w245:bool, "quality"=w244:i32)
                n163 = case "Link?" shown="False" w245 {
                  tunnel: w244 -> [w250 _]
                  tunnel: [w249 UtilityLib.valueStatus."no info available" ("valueStatus")] -> w247
                  tunnel: w246 -> [w248 _]
                  tunnel: [w248 w251] -> w242
                  frame False {
                    n164 = call "CoreLib.quality 2 status.vi"("quality"=w250) -> ("valueStatus"=w249:T4)  [unwired: 18 in]
                  }
                  frame True {
                    n165 = call "EmptyString.vi"() -> ("String"=w251:string)
                  }
                }
                n166 = Type Cast(type="" ("regular expression"), x=w242) -> (*(type *) &x=w241:string)
                n167 = String To Path(string=w241) -> (path=w238:path)
                n168 = control-ref of="SetFileLocation"() -> (w236:refnum<vi>)
                n169 = Build Path(base path=w238, name or relative path="MCP&PhosVolControl") -> (appended path=w239:path)
                n170 = property class="Path"(reference=w236, "Value"=w239) -> ()  [unwired: 1 in, 2 out]
                n171 = call "UtilityLib.set color of GUI object.vi"("GUI object Ref"=w236, "valueStatus"=w247) -> ()  [unwired: 17 in, 1 out]
              }
              frame #1 {
                # "Update Last Loaded File"
                n172 = control-ref of="Last Loaded File_Data"() -> (w254:refnum<vi>)
                n173 = control-ref of="SetFileLocation"() -> (w258:refnum<vi>)
                n174 = control-ref of="Last Loaded File"() -> (w257:refnum<vi>)
                n175 = property class="Clust (strict)"(reference=w254) -> ("Value"=w259:T5)  [unwired: 1 in, 2 out]
                n176 = call "LastLoadedFile.vi"("SetFileLocation"=w258, "Last Loaded File"=w257, "GUIName"="mcp&phosvol", "DIMControSet in"=w255, "SetValueInfo in"=w253, "NewVal"=w259) -> ()  [unwired: 14 in]
              }
            }
          }
          event Value Change {
            # "Update Last Loaded File"
            n177 = event-data() -> ("NewVal"=w264:T3)  [unwired: 1 in]
            n178 = control-ref of="SetFileLocation"() -> (w262:refnum<vi>)
            n179 = control-ref of="Last Loaded File"() -> (w261:refnum<vi>)
            n180 = call "LastLoadedFile.vi"("SetFileLocation"=w262, "Last Loaded File"=w261, "GUIName"="mcp&phosvol" ("string"), "DIMControSet in"=w263, "SetValueInfo in"=w260, "NewVal"=w264) -> ()  [unwired: 14 in]
          }
          event Value Change {
            n181 = event-data() -> ("CtlRef"=w267:refnum<vi>, "NewVal"=w270:T2)  [unwired: 1 in, 4 out]
            n182 = for "Check if Indicator Exists for the Monitor Value?" {
              tunnel: w270 -> [w279]
              tunnel: w269 -> [w276] mode=indexing
              tunnel: w267 -> [w275]
              # "Updating a Monitor Value"
              n183 = property class="DigNum (strict)"(reference=w276) -> (reference out=w271:refnum<vi>, "Label.Text"=w273:string)  [unwired: 1 in, 1 out]
              n184 = property class="Clust (strict)"(reference=w275) -> ("Label.Text"=w277:string)  [unwired: 1 in, 2 out]
              n185 = Match Pattern(string=w277, regular expression="Data") -> (before substring=w272:string)  [unwired: 1 in, 3 out]
              n186 = Equal?(x=w273, y=w272) -> (x = y?=w274:bool)
              n187 = case "Indicator exists?" shown="True" w274 {
                tunnel: w279 -> [w286 _]
                tunnel: w271 -> [w280 _]
                frame True {
                  n188 = Unbundle By Name(w286) -> ("data"=w282:dbl, "no link"=w283:bool, "quality"=w285:i32)
                  n189 = case shown="True" w283 {
                    tunnel: w285 -> [w289 _]
                    tunnel: [w288 UtilityLib.valueStatus."no info available" ("valueStatus")] -> w284
                    tunnel: w282 -> [w287 _]
                    tunnel: [w287 inf] -> w281
                    frame False {
                      n190 = call "CoreLib.quality 2 status.vi"("quality"=w289) -> ("valueStatus"=w288:T4)  [unwired: 18 in]
                    }
                    frame True {
                    }
                  }
                  n191 = property class="DigNum (strict)"(reference=w280, "Value"=w281) -> ()  [unwired: 1 in, 2 out]
                  n192 = call "TextColor.vi"("valueStatus"=w284, "reference"=w280) -> ()  [unwired: 10 in]
                }
                frame False {
                }
              }
            }
          }
          event Value Change {
            n193 = event-data() -> ("CtlRef"=w293:refnum<vi>, "NewVal"=w295:T2)  [unwired: 1 in, 4 out]
            n194 = for "Check if Indicator Exists for the Monitor Value?" {
              tunnel: w295 -> [w304]
              tunnel: w292 -> [w301] mode=indexing
              tunnel: w293 -> [w300]
              # "Find Monitor Value Index"
              # "Updating a Monitor Value"
              n195 = property class="Bool (strict)"(reference=w301) -> (reference out=w296:refnum<vi>, "Label.Text"=w298:string)  [unwired: 1 in, 1 out]
              n196 = property class="Clust (strict)"(reference=w300) -> ("Label.Text"=w302:string)  [unwired: 1 in, 2 out]
              n197 = Match Pattern(string=w302, regular expression="Data") -> (before substring=w297:string)  [unwired: 1 in, 3 out]
              n198 = Equal?(x=w298, y=w297) -> (x = y?=w299:bool)
              n199 = case "Indicator exists?" shown="True" w299 {
                tunnel: w304 -> [w315 _]
                tunnel: w296 -> [w306 _]
                frame True {
                  n200 = Unbundle By Name(w315) -> ("data"=w310:dbl, "no link"=w309:bool, "quality"=w314:i32)
                  n201 = Equal?(x=i16 -1, y=w310) -> (x = y?=w311:bool)
                  n202 = Or(x=w311, y=w309) -> (x .or. y?=w308:bool)
                  n203 = case shown="False" w309 {
                    tunnel: w314 -> [w321 _]
                    tunnel: [w320 UtilityLib.valueStatus."no info available" ("valueStatus")] -> w307
                    tunnel: w310 -> [w319 _]
                    tunnel: [w318 _] -> w313
                    frame False {
                      n204 = call "CoreLib.quality 2 status.vi"("quality"=w321) -> ("valueStatus"=w320:T4)  [unwired: 18 in]
                      n205 = Equal To 0?(x=w319) -> (x = 0?=w318:bool)
                    }
                    frame True {
                    }
                  }
                  n206 = case shown="False" w308 {
                    tunnel: [cluster{u32, u32}[] [{6618880, 6618880}, {1985280, 1985280}, {11245188, 10125428}] ("Colors [4]") cluster{u32, u32}[] [{12369084, 12369084}, {12369084, 12369084}, {11245188, 10125428}] ("Colors [4]")] -> w305
                    frame False {
                    }
                    frame True {
                    }
                  }
                  n207 = property class="Bool (strict)"(reference=w306, "Val(Sgnl)"=w313, "Colors [4]"=w305) -> ()  [unwired: 1 in, 2 out]
                  n208 = call "TextColor(bool).vi"("valueStatus"=w307, "Ref"=w306) -> ()  [unwired: 10 in]
                }
                frame False {
                }
              }
            }
          }
          event Value Change {
            n209 = event-data() -> ("CtlRef"=w325:refnum<vi>)  [unwired: 1 in]
            n210 = property on="FileUpToDate" class="Bool (strict)"() -> ("Value"=w323:bool)  [unwired: 2 in, 2 out]
            n211 = call "FileUpToDate.vi"("FileUpToDate in"=w323, "DIMControSet out"=w324, "CtlRef"=w325) -> ("FileUpToDate out"=w326:bool)  [unwired: 16 in]
            n212 = property on="FileUpToDate" class="Bool (strict)"("Value"=w326) -> ()  [unwired: 2 in, 2 out]
          }
          event "BOB3_Pho", "BOB3_MCP", "BOB5_Pho", "BOB5_MCP", "BOB6_Pho", "BOB6_MCP", "BOB1_Pho", "BOB1_MCP", "CEM_Plate", "Daly_Collector": Value Change {
            # "Find sub-panel index"
            # "opening or closing a sub-panel"
            n213 = event-data() -> ("CtlRef"=w328:refnum<vi>)  [unwired: 1 in]
            n214 = Search 1D Array(1D array=w329, element=w328) -> (index of element=w334:i32)  [unwired: 1 in]
            n215 = Index Array(array=w335, index=w334) -> (element=w332:refnum<vi>)
            n216 = invoke class="Bool" method="Reinit To Default"(reference=w328) -> ()  [unwired: 2 in, 3 out]
            n217 = property class="VI"(reference=w332) -> ("Front Panel.Open"=w331:bool)  [unwired: 1 in, 2 out]
            n218 = case "Panel Already Open?" shown="False" w331 {
              tunnel: w328 -> [w336 _]
              tunnel: w332 -> [_ w339]
              tunnel: [w337 refnum<vi> refnum ("vi reference")] -> w330
              frame False {
                n219 = call "OpenPanel.vi"("CtlRef"=w336) -> ("vi reference"=w337:refnum<vi>)  [unwired: 2 in]
              }
              frame True {
                n220 = call "PanelClose.vi"("vi reference"=w339) -> ()
              }
            }
            n221 = Replace Array Subset(array=w335, new element=w330, index=w334) -> (w333:refnum<vi>[])
          }
          event Timeout {
            # "Timeout"
            n222 = event-data() -> ()  [unwired: 1 in, 3 out]
          }
          event Panel Close? {
            n223 = event-data() -> ()  [unwired: 1 in, 1 out]
            n224 = stacked-sequence {
              tunnel: w345 -> [w351 _]
              tunnel: w344 -> [w350 _]
              tunnel: w343 -> [w349 _]
              tunnel: w342 -> [w348 _]
              tunnel: w341 -> [w353 _]
              frame #0 {
                # "Release DIM Services"
                n225 = for "For Each Service" {
                  tunnel: w348 -> [w355] mode=indexing
                  n226 = Not A Number/Path/Refnum?(number/path/refnum=w355) -> (NaN/Path/Refnum?=w354:bool)
                  n227 = case "Not a Reference?" shown="False" w354 {
                    tunnel: w355 -> [w356 _]
                    frame False {
                      n228 = call "DimIndicators.dic_release_service.vi"("controlRef"=w356) -> ()  [unwired: 18 in, 1 out]
                    }
                    frame True {
                    }
                  }
                }
                n229 = for "For Each Service" {
                  tunnel: w350 -> [w361] mode=indexing
                  n230 = Not A Number/Path/Refnum?(number/path/refnum=w361) -> (NaN/Path/Refnum?=w360:bool)
                  n231 = case "Not a Reference?" shown="False" w360 {
                    tunnel: w361 -> [w362 _]
                    frame False {
                      n232 = call "DimIndicators.dic_release_service.vi"("controlRef"=w362) -> ()  [unwired: 18 in, 1 out]
                    }
                    frame True {
                    }
                  }
                }
                n233 = for "Close Open Panels" {
                  tunnel: w353 -> [w366] mode=indexing
                  n234 = call "PanelClose.vi"("vi reference"=w366) -> ()
                }
                n235 = for "For Each Service" {
                  tunnel: w349 -> [w358] mode=indexing
                  n236 = Not A Number/Path/Refnum?(number/path/refnum=w358) -> (NaN/Path/Refnum?=w357:bool)
                  n237 = case "Not a Reference?" shown="False" w357 {
                    tunnel: w358 -> [w359 _]
                    frame False {
                      n238 = call "DimIndicators.dic_release_service.vi"("controlRef"=w359) -> ()  [unwired: 18 in, 1 out]
                    }
                    frame True {
                    }
                  }
                }
                n239 = for "For Each Service" {
                  tunnel: w351 -> [w364] mode=indexing
                  n240 = Not A Number/Path/Refnum?(number/path/refnum=w364) -> (NaN/Path/Refnum?=w363:bool)
                  n241 = case "Not a Reference?" shown="False" w363 {
                    tunnel: w364 -> [w365 _]
                    frame False {
                      n242 = call "DimIndicators.dic_release_service.vi"("controlRef"=w365) -> ()  [unwired: 18 in, 1 out]
                    }
                    frame True {
                    }
                  }
                }
                n243 = control-ref of="Last Loaded File_Data"() -> (w352:refnum<vi>)
                n244 = control-ref of="SetFileLocation_Data"() -> (w347:refnum<vi>)
                n245 = call "DimIndicators.dic_release_service.vi"("controlRef"=w352) -> ()  [unwired: 18 in, 1 out]
                n246 = call "DimIndicators.dic_release_service.vi"("controlRef"=w347) -> ()  [unwired: 18 in, 1 out]
              }
              frame #1 {
                # "Close Front Panel"
                n247 = Current VI's Path() -> (path=w370:path)
                n248 = Open VI Reference(vi path=w370) -> (vi reference=w368:refnum<vi>, error out=w367:errorcluster)  [unwired: 5 in]
                n249 = property class="VI"(reference=w368, error in=w367, "Front Panel Window:Open"=FALSE) -> ()  [unwired: 2 out]
              }
            }
            n250 = event-data() -> ()  [unwired: 2 in, 1 out]
          }
        }
      }
    }
    frame #3 {
      n251 = stacked-sequence {
        tunnel: w375 -> [w378 _ _]
        tunnel: w374 -> [w382 _ _]
        tunnel: w373 -> [w379 _ _]
        tunnel: w372 -> [w380 _ _]
        tunnel: w371 -> [w377 _ _]
        frame #0 {
          # "Release DIM Services"
          n252 = control-ref of="Last Loaded File_Data"() -> (w381:refnum<vi>)
          n253 = control-ref of="SetFileLocation_Data"() -> (w376:refnum<vi>)
          n254 = call "DimIndicators.dic_release_service.vi"("controlRef"=w381) -> ()  [unwired: 18 in, 1 out]
          n255 = call "DimIndicators.dic_release_service.vi"("controlRef"=w376) -> ()  [unwired: 18 in, 1 out]
          n256 = for "For Each Service" {
            tunnel: w377 -> [w384] mode=indexing
            n257 = Not A Number/Path/Refnum?(number/path/refnum=w384) -> (NaN/Path/Refnum?=w383:bool)
            n258 = case "Not a Reference?" shown="False" w383 {
              tunnel: w384 -> [w385 _]
              frame False {
                n259 = call "DimIndicators.dic_release_service.vi"("controlRef"=w385) -> ()  [unwired: 18 in, 1 out]
              }
              frame True {
              }
            }
          }
          n260 = for "For Each Service" {
            tunnel: w379 -> [w390] mode=indexing
            n261 = Not A Number/Path/Refnum?(number/path/refnum=w390) -> (NaN/Path/Refnum?=w389:bool)
            n262 = case "Not a Reference?" shown="False" w389 {
              tunnel: w390 -> [w391 _]
              frame False {
                n263 = call "DimIndicators.dic_release_service.vi"("controlRef"=w391) -> ()  [unwired: 18 in, 1 out]
              }
              frame True {
              }
            }
          }
          n264 = for "For Each Service" {
            tunnel: w380 -> [w393] mode=indexing
            n265 = Not A Number/Path/Refnum?(number/path/refnum=w393) -> (NaN/Path/Refnum?=w392:bool)
            n266 = case "Not a Reference?" shown="False" w392 {
              tunnel: w393 -> [w394 _]
              frame False {
                n267 = call "DimIndicators.dic_release_service.vi"("controlRef"=w394) -> ()  [unwired: 18 in, 1 out]
              }
              frame True {
              }
            }
          }
          n268 = for "For Each Service" {
            tunnel: w378 -> [w387] mode=indexing
            n269 = Not A Number/Path/Refnum?(number/path/refnum=w387) -> (NaN/Path/Refnum?=w386:bool)
            n270 = case "Not a Reference?" shown="False" w386 {
              tunnel: w387 -> [w388 _]
              frame False {
                n271 = call "DimIndicators.dic_release_service.vi"("controlRef"=w388) -> ()  [unwired: 18 in, 1 out]
              }
              frame True {
              }
            }
          }
          n272 = for "Close Open Panels" {
            tunnel: w382 -> [w395] mode=indexing
            n273 = call "PanelClose.vi"("vi reference"=w395) -> ()
          }
        }
        frame #1 {
          # "Close Front Panel"
          n274 = Current VI's Path() -> (path=w399:path)
          n275 = Open VI Reference(vi path=w399) -> (vi reference=w397:refnum<vi>, error out=w396:errorcluster)  [unwired: 5 in]
          n276 = property class="VI"(reference=w397, error in=w396, "Front Panel Window:Open"=FALSE) -> ()  [unwired: 2 out]
        }
        frame #2 {
          # "Stop Panel"
          n277 = Stop(stop? (T)=TRUE) -> ()
        }
      }
    }
  }
  n278 = call "LVDimInterface.dim_operate.vi"("DNSNode"="lebit-balcony" ("DNS node")) -> ()  [unwired: 19 in]
